vi "Result.Parse Data File Name to SN, Time, Result, Flex FTS.vi"(11 "File Path":path) -> (1 "DateTime":timestamp, 2 "SN":string)   [LabVIEW 2019]
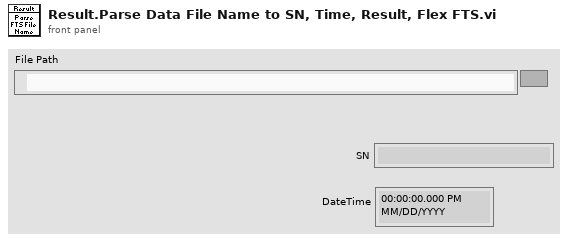
[diagram p1: front panel]
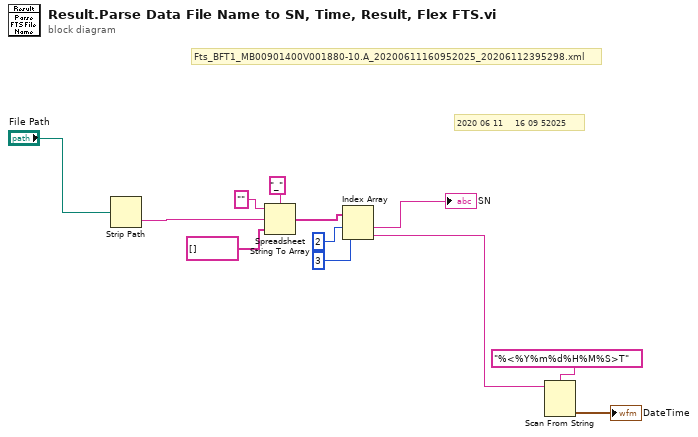
[diagram p0: block diagram]
diagram:
  # "2020 06 11    16 09 52025"
  # "Fts_BFT1_MB00901400V001880-10.A_20200611160952025_20206112395298.xml"
  n1 = Strip Path(path="File Path") -> (name=w9:string)  [unwired: 1 out]
  n2 = Spreadsheet String To Array(delimiter (Tab)="_", format string="", spreadsheet string=w9, array type (2D Dbl)=string[] []) -> (array=w5:string[])
  n3 = Index Array(array=w5, index #1=2 ("index"), index #2=3 ("index")) -> (element #1=→"SN":string, element #2=w3:string)
  n4 = Scan From String(format string="%<%Y%m%d%H%M%S>T", input string=w3) -> (output 1=→"DateTime":timestamp)  [unwired: 3 in, 3 out]
